vi "Auto Shoot Using Dashboard Data.vi"(0 "Auto Preparation for Shooting":bool, 1 "Pilot X":dbl, 2 "Pilot Y":dbl, 3 "Elevation":dbl, 4 "Shoot Motors":dbl, 5 "Le Fire At Will":bool, 6 "Camera Centered?":bool, 7 "ReCenterize":bool, 8 "Stop Centerizing":bool, 9 "Fine Tune":bool, 10 "Stop Angle Adjust":bool, 12 "Cam offset - Delta X %":dbl, 13 "override \"Ready to Fire\"":bool) -> (15 "X Drive Arcade":dbl, 18 "Y Drive Arcade":dbl, 19 "Ready to Fire!":bool)   [LabVIEW 2012]
uses:
  Motors Values.vi
  BotStatus.vi
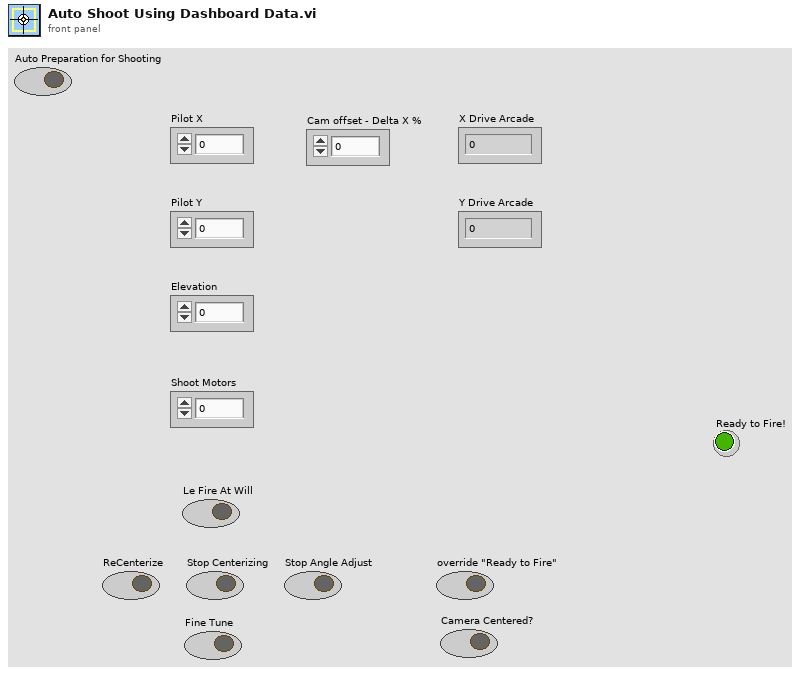
[diagram p1: front panel]
types:
  T1 = cluster{"Target Position X":dbl, "Target Position Y":dbl, "Target Found":bool}
  T2 = typedef "WPI_EncoderDevRef.ctl" = cluster{"DevStatus":errorcluster, "EncoderIndex":T3, "CounterIndex":T4, "DistancePerCount":dbl, "Decoding Type":T5}
  T3 = typedef "FPGA_EncoderIdx.ctl" = enum8{"Enc 0", "Enc 1", "Enc 2", "Enc 3", "Invalid"}
  T4 = typedef "FPGA_CounterCtrSystemIndex.ctl" = enum8{"Ctr 0", "Ctr 1", "Ctr 2", "Ctr 3", "Ctr 4", "Ctr 5", "Ctr 6", "Ctr 7", "Invalid"}
  T5 = typedef "WPI_EncoderType.ctl" = enum16{"1x", "2x", "4x"}
  T6 = cluster{"Middle":bool, "InCannon":bool, "InFlipper":bool, "FlipperAtPlace":bool, "Bottom":bool, "FrisbeeDirection":bool}
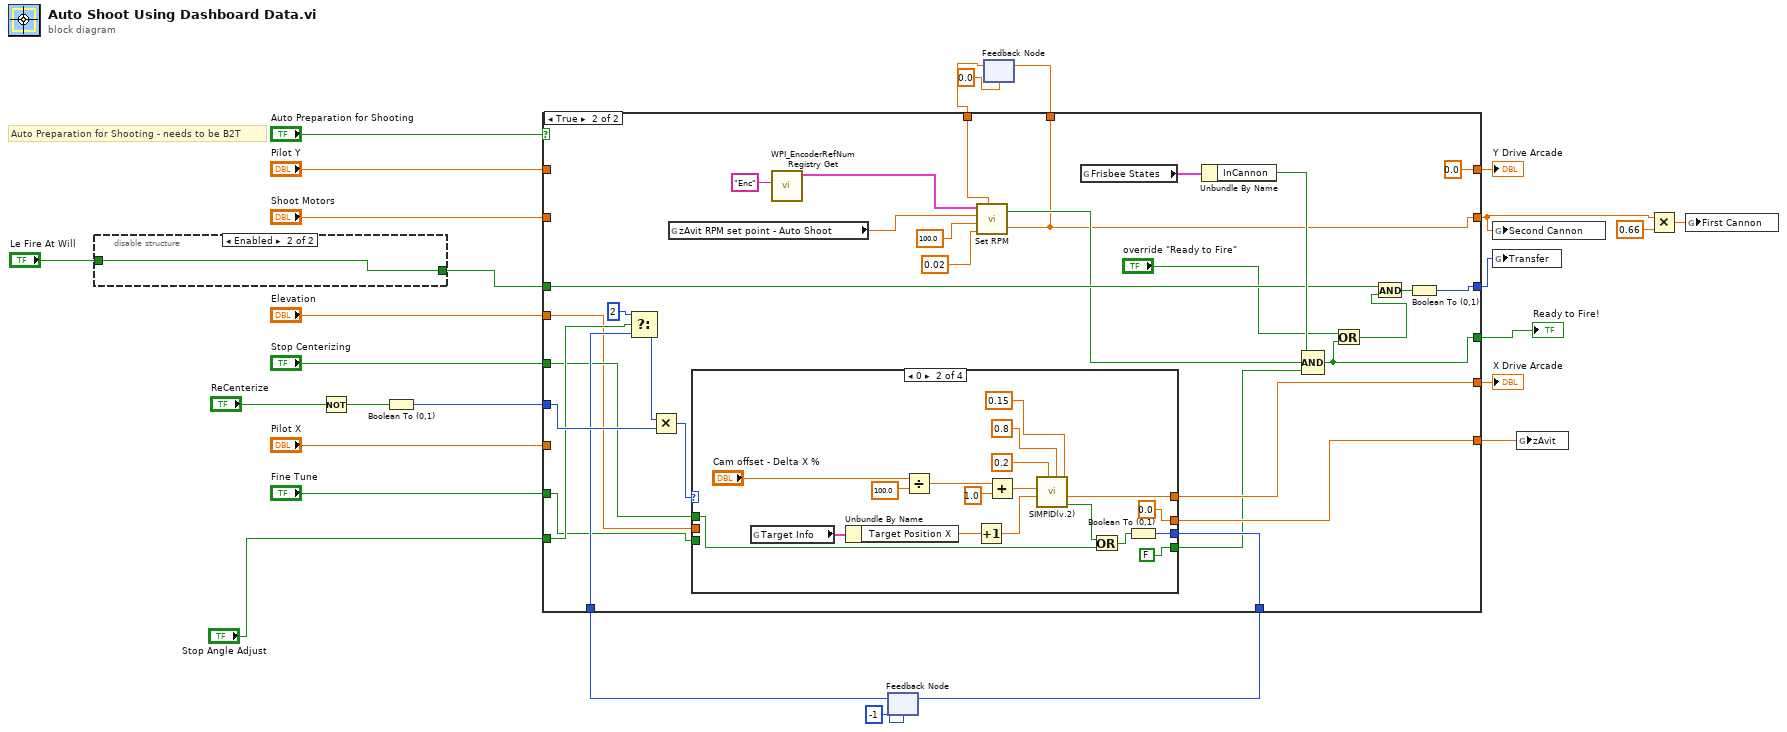
[diagram p0: block diagram]
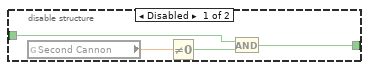
[diagram p2: hidden frame]
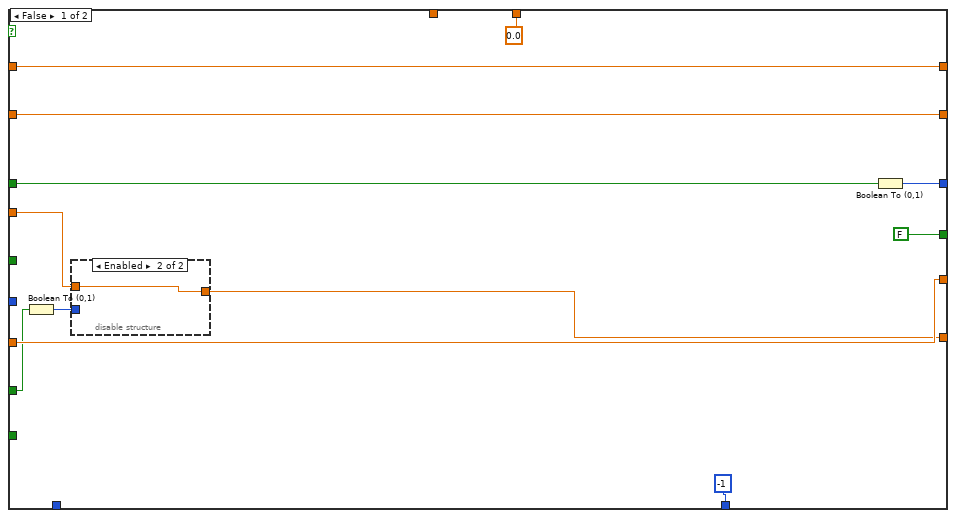
[diagram p3: hidden frame]
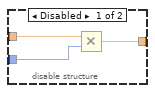
[diagram p4: hidden frame]
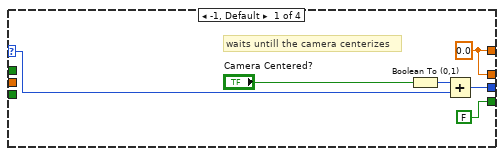
[diagram p5: hidden frame]
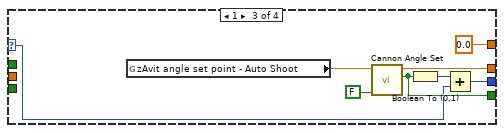
[diagram p6: hidden frame]
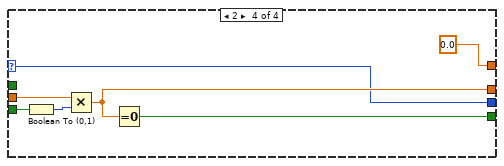
[diagram p7: hidden frame]
diagram:
  # "Auto Preparation for Shooting - needs to be B2T"
  n1 = disable-structure shown="Enabled" {
    disable-tunnel: "Le Fire At Will" -> [w29 w32]
    disable-tunnel: [w28 w32] -> w13
    frame Disabled {
      n2 = global read "Motors Values.vi" "Second Cannon"() -> (w31:dbl)
      n3 = Not Equal To 0?(x=w31) -> (x != 0?=w30:bool)
      n4 = And(x=w29, y=w30) -> (x .and. y?=w28:bool)
    }
    frame Enabled {
    }
  }
  n5 = Not(x="ReCenterize") -> (.not. x?=w9:bool)
  n6 = Boolean To (0,1)(Boolean=w9) -> (0, 1=w8:i16)
  n7 = feedback #1(-1) -> (w6:i32)
  n8 = feedback #2(0.0 ("Vbus Out")) -> (w2:dbl)
  n9 = case shown="True" "Auto Preparation for Shooting" {
    tunnel: [w39 w56] -> w24
    tunnel: [w44 w57] -> w25
    tunnel: "Pilot X" -> [w44 _]
    tunnel: "Elevation" -> [w43 w52]
    tunnel: w13 -> [w37 w73]
    tunnel: [w42 w76] -> w22
    tunnel: [w41 w50] -> w19
    tunnel: "Shoot Motors" -> [w41 _]
    tunnel: "Pilot Y" -> [w40 _]
    tunnel: [w40 0.0] -> w16
    tunnel: [FALSE w69] -> w15
    tunnel: "Fine Tune" -> [w35 w51]
    tunnel: "Stop Centerizing" -> [_ w53]
    tunnel: w8 -> [_ w70]
    tunnel: w6 -> [_ w66]
    tunnel: [-1 w58] -> w5
    tunnel: "Stop Angle Adjust" -> [_ w54]
    tunnel: [0.0 ("Vbus Out") w50] -> w3
    tunnel: w2 -> [_ w49]
    frame False {
      n10 = Boolean To (0,1)(Boolean=w35) -> (0, 1=w38:i16)
      n11 = disable-structure shown="Enabled" {
        disable-tunnel: w43 -> [w47 w48]
        disable-tunnel: [w46 w48] -> w39
        disable-tunnel: w38 -> [w45 _]
        frame Disabled {
          n12 = Multiply(x=w47, y=w45) -> (x*y=w46:dbl)
        }
        frame Enabled {
        }
      }
      n13 = Boolean To (0,1)(Boolean=w37) -> (0, 1=w42:i16)
    }
    frame True {
      n14 = Select(t=2, s=w54, f=w66) -> (s? t:f=w71:i32)
      n15 = Multiply(x=w71, y=w70) -> (x*y=w59:i32)
      n16 = global read "BotStatus.vi" "zAvit RPM set point - Auto Shoot"() -> (w63:dbl)
      n17 = case shown="0" w59 {
        selector: w59 -> [w82 _ w104 w113]
        tunnel: [w79 w95 0.0 ("Pilot X") 0.0 ("Pilot X")] -> w57
        tunnel: [w81 w94 w103 w113] -> w58
        tunnel: [w79 0.0 ("zAvit Vbus Out") w109 w114] -> w56
        tunnel: [FALSE ("On Target") FALSE ("On Target") w105 w115] -> w55
        tunnel: w53 -> [_ w85 _ _]
        tunnel: w52 -> [_ _ _ w116]
        tunnel: w51 -> [_ _ _ w111]
        frame -1, Default {
          w79 = 0.0 ("Pilot X")
          # "waits untill the camera centerizes"
          n18 = Boolean To (0,1)(Boolean="Camera Centered?") -> (0, 1=w83:i16)
          n19 = Add(x=w83, y=w82) -> (x+y=w81:i32)
        }
        frame 0 {
          n20 = global read "BotStatus.vi" "Target Info"() -> (w97:T1)
          n21 = Unbundle By Name(w97) -> ("Target Position X"=w96:dbl)
          n22 = Divide(x="Cam offset - Delta X %", y=100.0) -> (x/y=w89:dbl)
          n23 = Increment(x=w96) -> (x+1=w101:dbl)
          n24 = Add(x=w89, y=1.0 ("Set Point")) -> (x+y=w90:dbl)
          n25 = call "SIMPID(v.2).vi"("Range"=0.15, "upper limit"=0.8, "lower limit"=0.2, "Current Point"=w101, "Set Point"=w90) -> ("On Target"=w87:bool, "result"=w95:dbl)  [unwired: 5 in]
          n26 = Or(x=w87, y=w85) -> (x .or. y?=w86:bool)
          n27 = Boolean To (0,1)(Boolean=w86) -> (0, 1=w94:i16)
        }
        frame 1 {
          n28 = global read "BotStatus.vi" "zAvit angle set point - Auto Shoot"() -> (w110:dbl)
          n29 = call "Cannon Angle Set.vi"("set angle 0 to be min angle"=FALSE, "Angle Set Point"=w110) -> ("On Target"=w105:bool, "zAvit Vbus Out"=w109:dbl)  [unwired: 8 in]
          n30 = Boolean To (0,1)(Boolean=w105) -> (0, 1=w106:i16)
          n31 = Add(x=w106, y=w104) -> (x+y=w103:i32)
        }
        frame 2 {
          n32 = Boolean To (0,1)(Boolean=w111) -> (0, 1=w117:i16)
          n33 = Multiply(x=w116, y=w117) -> (x*y=w114:dbl)
          n34 = Equal To 0?(x=w114) -> (x = 0?=w115:bool)
        }
      }
      n35 = call <vilib>:"WPI_EncoderRefNum Registry Get.vi"("refnum name"="Enc") -> ("EncoderDevRef"=w64:T2)  [unwired: 9 in, 1 out]
      n36 = call "Set RPM.vi"("EncoderDevRef"=w64, "Set Point RPM"=w63, "Range RPM"=100.0, "Gain Vbus"=0.02, "Previous Vbus"=w49) -> ("READY!"=w60:bool, "Vbus Out"=w50:dbl)
      n37 = global read "BotStatus.vi" "Frisbee States"() -> (w78:T6)
      n38 = Unbundle By Name(w78) -> ("InCannon"=w77:bool)
      n39 = Compound Arithmetic op=AND(w77, w60, w55) -> (w69:bool)
      n40 = Or(x="override \"Ready to Fire\"", y=w69) -> (x .or. y?=w67:bool)
      n41 = And(x=w73, y=w67) -> (x .and. y?=w74:bool)
      n42 = Boolean To (0,1)(Boolean=w74) -> (0, 1=w76:i16)
    }
  }
  "X Drive Arcade" <- w25
  "Y Drive Arcade" <- w16
  "Ready to Fire!" <- w15
  n43 = feedback-in #1(w5) -> ()
  n44 = feedback-in #2(w3) -> ()
  n45 = global write "Motors Values.vi" "Second Cannon"(w19) -> ()
  n46 = global write "Motors Values.vi" "Transfer"(w22) -> ()
  n47 = global write "Motors Values.vi" "zAvit"(w24) -> ()
  n48 = Multiply(x=w19, y=0.66) -> (x*y=w20:dbl)
  n49 = global write "Motors Values.vi" "First Cannon"(w20) -> ()
